vi "Select Inteleaved Channels.vi"(9 "Boolean selection 1D":bool[](array[boolean]), 10 "Total channels":i32=2, 11 "Input":i16[](array[numeric])=[1, 11, 21, 31, 2, 12, 22, 32, 3, 13, 23, 33]) -> (3 "Output":i16[][](array[numeric])=[[1, 11, 21, 31, 2, 12, 22, 32, 3, 13, 23, 33]])   [LabVIEW 2024]
panel:
  out "Input 3":i16[][](array[numeric])
  in  "Num elements":i32[](array[numeric])
  in  "Input 2":i16[](array[numeric])=[41, 51, 42, 52, 43, 53]
  out "Array":i32[](array[numeric])
  in  "Channels to keep":i32[](array[numeric])
  out "element":i32
  out "appended array 3":i16[][](array[numeric])
  out "appended array 2":i16[][](array[numeric])
  out "appended array":i16[][](array[numeric])
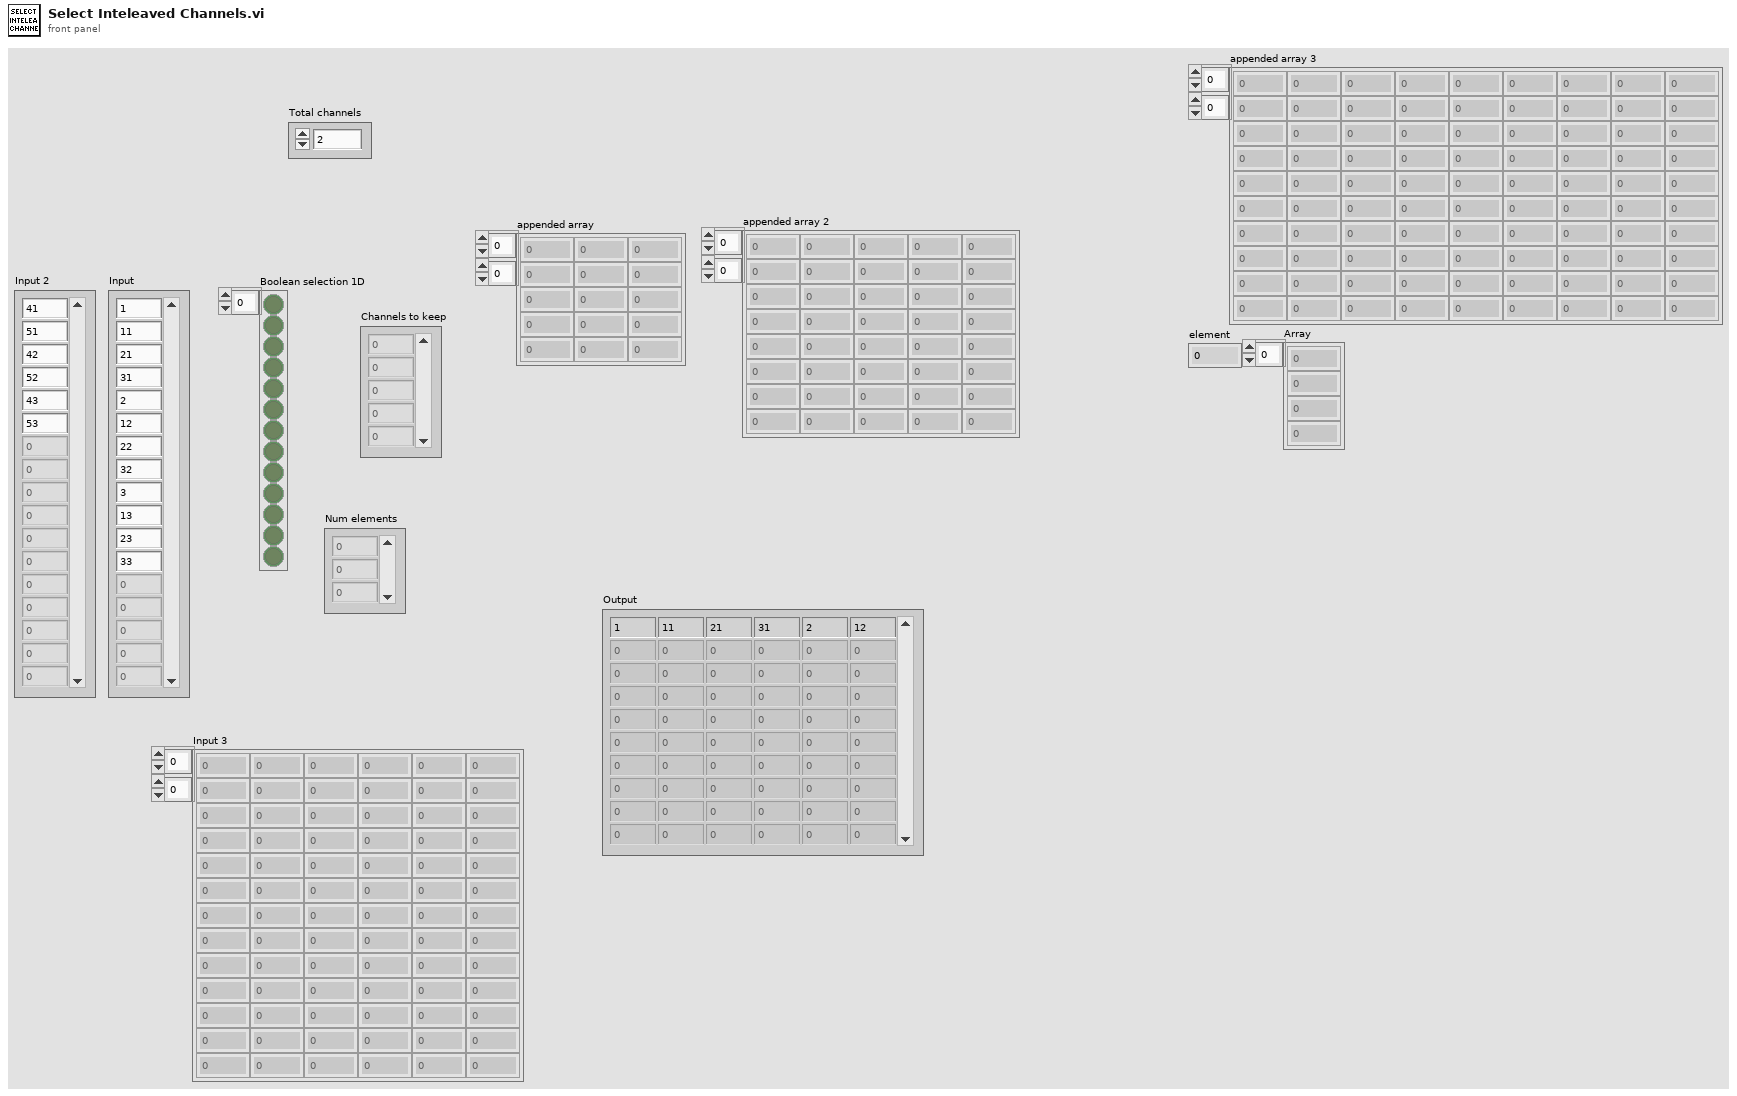
[diagram p1: front panel]
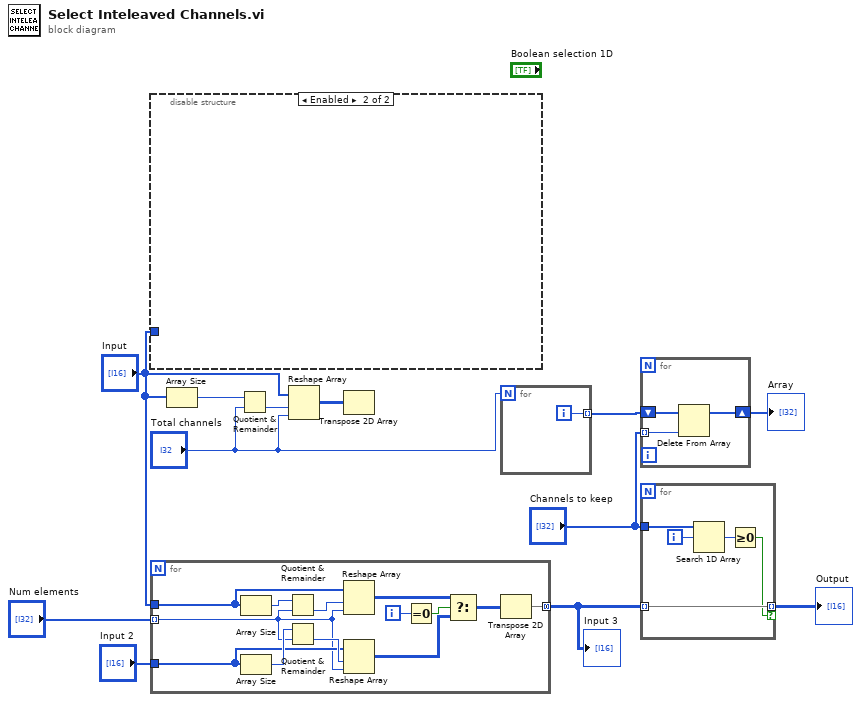
[diagram p0: block diagram]
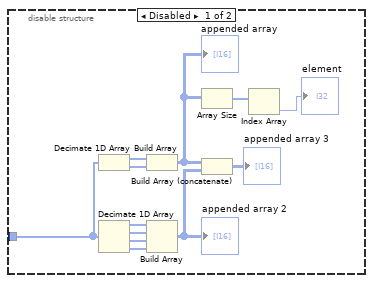
[diagram p2: hidden frame]
diagram:
  n1 = disable-structure shown="Enabled" {
    disable-tunnel: "Input" -> [w18 _]
    frame Disabled {
      n2 = Decimate 1D Array(w18) -> (w24:i16[], w23:i16[])
      n3 = Decimate 1D Array(w18) -> (w22:i16[], w21:i16[], w20:i16[], w19:i16[])
      n4 = Build Array(w24, w23) -> (w14:i16[][])
      "appended array" <- w14
      n5 = Build Array(w22, w21, w20, w19) -> (w17:i16[][])
      "appended array 2" <- w17
      n6 = Array Size(array=w14) -> (size(s)=w15:i32[])
      n7 = Build Array (concatenate)(w14, w17) -> (→"appended array 3":i16[][])
      n8 = Index Array(array=w15) -> (element=→"element":i32)  [unwired: 1 in]
    }
    frame Enabled {
    }
  }
  n9 = for {
    tunnel: "Num elements" -> [w30] mode=indexing
    tunnel: "Input" -> [w34]
    tunnel: "Input 2" -> [w31]
    tunnel: [w25] -> w1 mode=concatenating
    i -> [w37]
    n10 = Array Size(array=w34) -> (size(s)=w36:i32)
    n11 = Array Size(array=w31) -> (size(s)=w32:i32)
    n12 = Quotient & Remainder(x=w36, y=w30) -> (floor(x/y)=w35:i32)  [unwired: 1 out]
    n13 = Quotient & Remainder(x=w32, y=w30) -> (floor(x/y)=w33:i32)  [unwired: 1 out]
    n14 = Reshape Array(w34, w35, w30) -> (w28:i16[][])
    n15 = Reshape Array(w31, w33, w30) -> (w27:i16[][])
    n16 = Equal To 0?(x=w37) -> (x = 0?=w29:bool)
    n17 = Select(t=w28, s=w29, f=w27) -> (s? t:f=w26:i16[][])
    n18 = Transpose 2D Array(2D array=w26) -> (transposed array=w25:i16[][])
  }
  "Input 3" <- w1
  n19 = Array Size(array="Input") -> (size(s)=w11:i32)
  n20 = Quotient & Remainder(x=w11, y="Total channels") -> (floor(x/y)=w12:i32)  [unwired: 1 out]
  n21 = Reshape Array("Input", w12, "Total channels") -> (w9:i16[][])
  n22 = Transpose 2D Array(2D array=w9) -> ()  [unwired: 1 out]
  n23 = for {
    N: "Total channels" -> [_]
    tunnel: [w38] -> w7 mode=indexing
    i -> [w38]
  }
  n24 = for {
    tunnel: "Channels to keep" -> [w40] mode=indexing
    shift-right: [w39] -> w6
    shift-left: w7 -> [w41]
    n25 = Delete From Array(array=w41, index=w40) -> (array with subset deleted=w39:i32[])  [unwired: 1 in, 1 out]
  }
  "Array" <- w6
  n26 = for {
    tunnel: w1 -> [w46] mode=indexing
    tunnel: [w46] -> w10 mode=indexing if=w42
    tunnel: "Channels to keep" -> [w44]
    i -> [w43]
    n27 = Search 1D Array(1D array=w44, element=w43) -> (index of element=w45:i32)  [unwired: 1 in]
    n28 = Greater Or Equal To 0?(x=w45) -> (x >= 0?=w42:bool)
  }
  "Output" <- w10
